vi "GPS_PositionChangeEventExe.vi"(0 "Devices In":u64[](array[numeric]), 1 "Event Registration Refnum In":refnum<event-registration>, 5 "error in (no error)":errorcluster) -> (10 "Index":i32, 12 "Event?":bool, 13 "phid":u64, 14 "Devices Out":u64[](array[numeric]), 15 "Event Registration Refnum Out":refnum<event-registration>, 16 "Latitude":dbl, 17 "Longitude":dbl, 18 "Altitude":dbl, 19 "error out":errorcluster)   [LabVIEW 2012, in "Phidget GPS.lvlib"]
doc: "${PositionChange:Header}"
uses:
  <instrlib>/Phidgets/Phidget GPS/Phidget GPS.lvlib
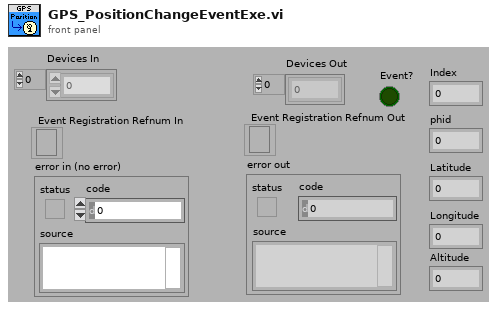
[diagram p1: front panel]
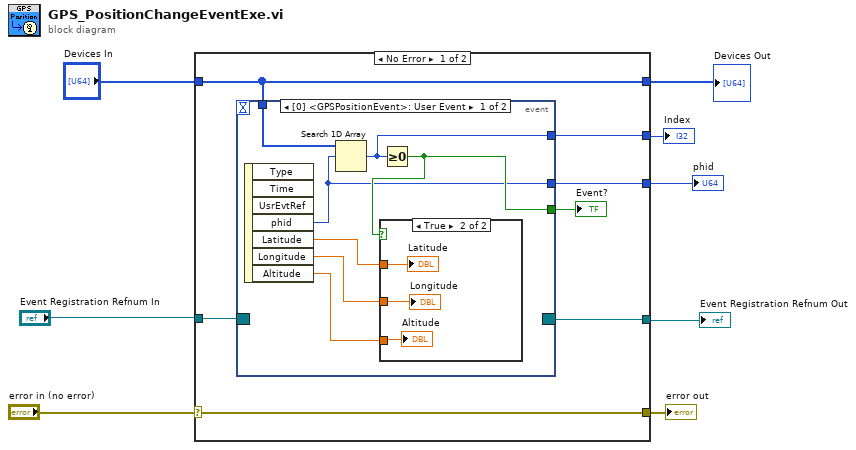
[diagram p0: block diagram]
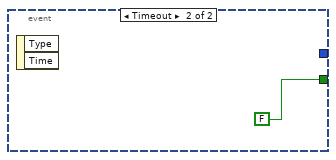
[diagram p3: hidden frame]
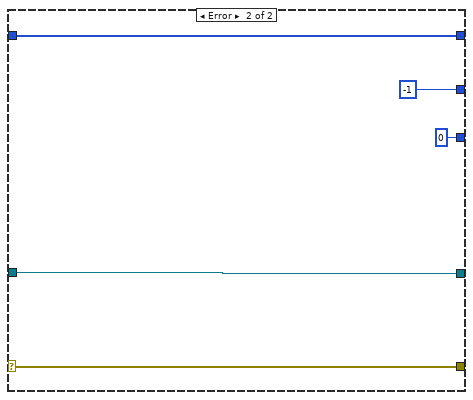
[diagram p4: hidden frame]
diagram:
  n1 = case shown="No Error" "error in (no error)" {
    selector: "error in (no error)" -> [w12 w31]
    tunnel: [w12 w31] -> w7
    tunnel: [w15 w30] -> w2
    tunnel: "Event Registration Refnum In" -> [w14 w30]
    tunnel: [w11 w29] -> w5
    tunnel: "Devices In" -> [w11 w29]
    tunnel: [w10 -1] -> w4
    tunnel: [w9 u64 0 ("phid")] -> w3
    frame No Error {
      n2 = event shown="[0] <GPSPositionEvent>: User Event" {
        selector: w14 -> [_ _]
        dyn-events: [_ _] -> w15
        timeout: _ -> [_ _]
        tunnel: [w21 FALSE] -> w13
        tunnel: w11 -> [w22 _]
        tunnel: [w20 _] -> w10
        tunnel: [w19 _] -> w9
        event User Event {
          n3 = event-data() -> ("phid"=w19:u64, "Latitude"=w18:dbl, "Longitude"=w17:dbl, "Altitude"=w16:dbl)  [unwired: 1 in, 3 out]
          n4 = Search 1D Array(1D array=w22, element=w19) -> (index of element=w20:i32)  [unwired: 1 in]
          n5 = Greater Or Equal To 0?(x=w20) -> (x >= 0?=w21:bool)
          n6 = case shown="True" w21 {
            tunnel: w18 -> [_ w25]
            tunnel: w17 -> [_ w24]
            tunnel: w16 -> [_ w23]
            frame False {
            }
            frame True {
              "Latitude" <- w25
              "Longitude" <- w24
              "Altitude" <- w23
            }
          }
        }
        event Timeout {
          n7 = event-data() -> ()  [unwired: 1 in, 2 out]
        }
      }
      "Event?" <- w13
    }
    frame Error {
    }
  }
  "error out" <- w7
  "Devices Out" <- w5
  "Index" <- w4
  "phid" <- w3
  "Event Registration Refnum Out" <- w2
